vi "Read Config String.vi"(8 "error in (no error)":errorcluster, 11 "Tag in":refnum<class "Tag.lvclass">) -> (0 "error out":errorcluster, 2 "Config String":string, 3 "Tag out":refnum<class "Tag.lvclass">)   [LabVIEW 2020, in "Tag Engine Core.lvlib" / "Tag.lvclass"]
doc: "_SubVI_"
uses:
  Tag.lvclass
  Tag.lvclass/Tag.ctl
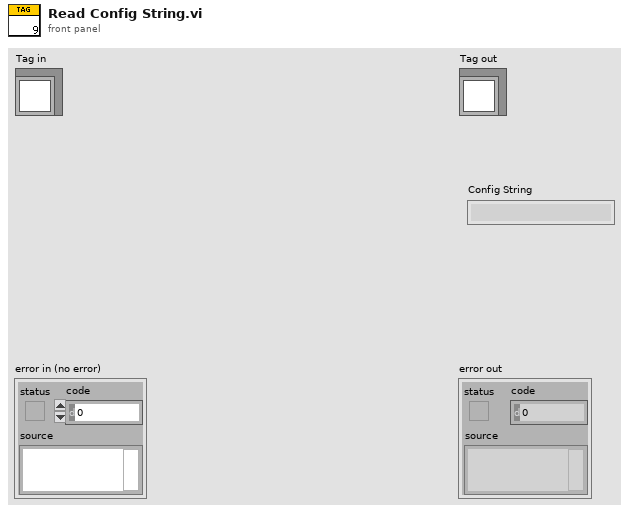
[diagram p1: front panel]
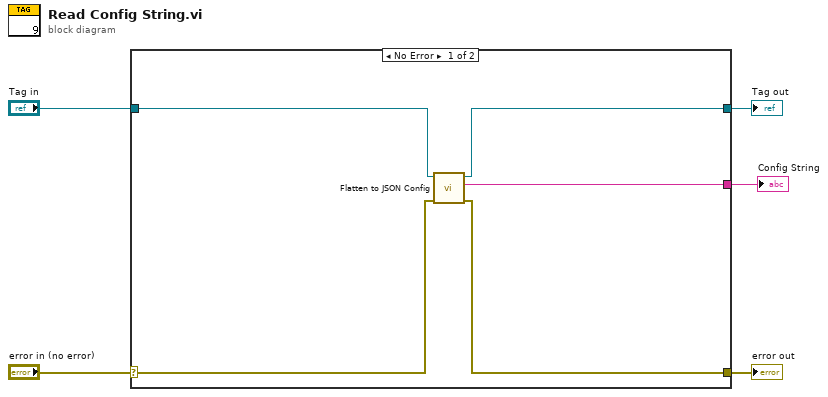
[diagram p0: block diagram]
diagram:
  n1 = case shown="No Error" "error in (no error)" {
    selector: "error in (no error)" -> [w8 w12]
    tunnel: [w7 w12] -> w4
    tunnel: [w10 w11] -> w2
    tunnel: "Tag in" -> [w9 w11]
    tunnel: [w6 _] -> w1
    frame No Error {
      n2 = call "Flatten to JSON Config.vi"("error in (no error)"=w8, "Tag in"=w9) -> ("error out"=w7:errorcluster, "JSON String"=w6:string, "Tag out"=w10:refnum<class "Tag.lvclass">)  [unwired: 7 in]
    }
    frame Error {
    }
  }
  "error out" <- w4
  "Tag out" <- w2
  "Config String" <- w1
